vi "XW_Map_E1E2_to_UV_PN.vi"(6 "Trimmed down TreeNode array":T1[](array[typedef]), 8 "Triangulated XW Calib Map Mesh":T2[](array[typedef]), 9 "(E2 / G2) + O2 (Volts)":dbl, 11 "(E1 / G1) + O1 (Volts)":dbl) -> (1 "V (m/s)":dbl=nan, 2 "U (m/s)":dbl=nan, 3 "Voltages are inside calibrated region":bool, 5 "Indices of traversed treenodes":i32[](array[numeric]), 7 "Indices of triangle array to test fully":i32[](array[numeric]))   [LabVIEW 2010]
uses:
  Triangle2D.ctl
  Qtree vis/Trimmed down TreeNode2D.ctl
panel:
  # "Paul Nathan 12/12/09\n\n09/03/10: Modified to use trimmed down\ntreenode array to reduce memory usage\nand increase speed"
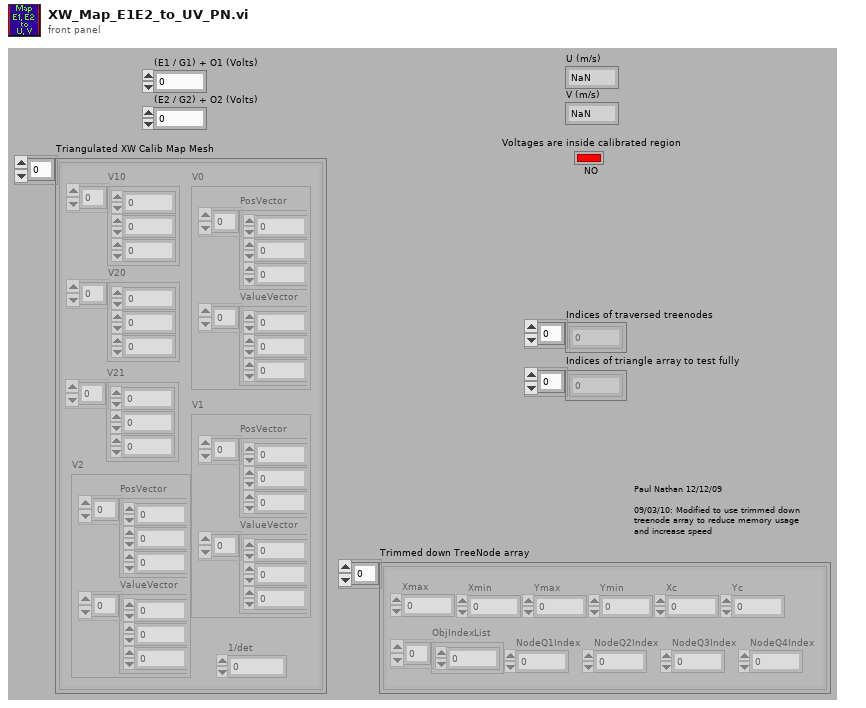
[diagram p1: front panel]
types:
  T1 = typedef "Trimmed down TreeNode2D.ctl" = cluster{"Xmax":dbl, "Xmin":dbl, "Ymax":dbl, "Ymin":dbl, "Xc":dbl, "Yc":dbl, "ObjIndexList":i32[], "NodeQ1Index":i32, "NodeQ2Index":i32, "NodeQ3Index":i32, "NodeQ4Index":i32}
  T2 = typedef "Triangle2D.ctl" = cluster{"V10":dbl[], "V20":dbl[], "1/det":dbl, "V0":cluster{"PosVector":dbl[], "ValueVector":dbl[]}, "V1":cluster{"PosVector":dbl[], "ValueVector":dbl[]}, "V2":cluster{"PosVector":dbl[], "ValueVector":dbl[]}, "V21":dbl[]}
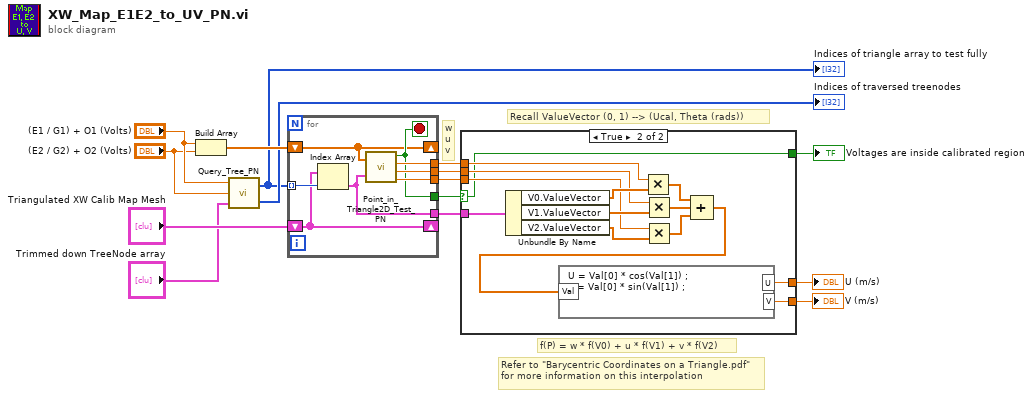
[diagram p0: block diagram]
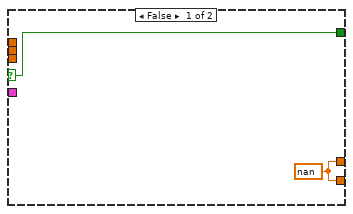
[diagram p2: hidden frame]
diagram:
  # "f(P) = w * f(V0) + u * f(V1) + v * f(V2)"
  # "Recall ValueVector (0, 1) --> (Ucal, Theta (rads))"
  # "Refer to \"Barycentric Coordinates on a Triangle.pdf\" for more information on this interpolation"
  # "w\nu\nv"
  n1 = Build Array("(E1 / G1) + O1 (Volts)", "(E2 / G2) + O2 (Volts)") -> (w6:dbl[])
  n2 = call "Query_Tree_PN.vi"("Trimmed down TreeNode array"="Trimmed down TreeNode array", "Query Y"="(E2 / G2) + O2 (Volts)", "Query X"="(E1 / G1) + O1 (Volts)") -> ("Indices of traversed treenodes"=→"Indices of traversed treenodes":i32[], "Indices of triangle array to test fully"=w2:i32[])
  "Indices of triangle array to test fully" <- w2
  n3 = for {
    tunnel: [w23] -> w14
    tunnel: [w22] -> w13
    tunnel: [w21] -> w12
    tunnel: [w18] -> w15
    tunnel: [w20] -> w11
    tunnel: w2 -> [w19] mode=indexing
    shift-right: [w17] -> _
    shift-left: "Triangulated XW Calib Map Mesh" -> [w17]
    shift-right: [w16] -> _
    shift-left: w6 -> [w16]
    stop <- w20 stop-if-true
    n4 = Index Array(array=w17, index=w19) -> (element=w18:T2)
    n5 = call "Point_in_Triangle2D_Test_PN.vi"("2D Point to Test"=w16, "Triangle2D"=w18) -> ("Point is in triangle"=w20:bool, "w"=w23:dbl, "u"=w22:dbl, "v"=w21:dbl)
  }
  n6 = case shown="True" w11 {
    selector: w11 -> [w25 w29]
    tunnel: w15 -> [_ w39]
    tunnel: w14 -> [_ w38]
    tunnel: w13 -> [_ w36]
    tunnel: w12 -> [_ w34]
    tunnel: [w25 w29] -> w10
    tunnel: [w24 w28] -> w9
    tunnel: [w24 w27] -> w8
    frame False {
      w24 = nan
    }
    frame True {
      n7 = Unbundle By Name(w39) -> ("V0.ValueVector"=w37:dbl[], "V1.ValueVector"=w35:dbl[], "V2.ValueVector"=w33:dbl[])
      n8 = Multiply(x=w38, y=w37) -> (x*y=w32:dbl[])
      n9 = Multiply(x=w36, y=w35) -> (x*y=w31:dbl[])
      n10 = Multiply(x=w34, y=w33) -> (x*y=w30:dbl[])
      n11 = Compound Arithmetic op=ADD(w32, w31, w30) -> (w26:dbl[])
      n12 = formula code="U = Val[0] * cos(Val[1]) ;\nV = Val[0] * sin(Val[1]) ;"("Val"=w26) -> ("U"=w28:dbl, "V"=w27:dbl)
    }
  }
  "U (m/s)" <- w9
  "V (m/s)" <- w8
  "Voltages are inside calibrated region" <- w10
